vi "Dash Bools.vi"(1 "Input":cluster{"Arm Safety":bool, "Arm Limit":bool}, 2 "Menu":T1) -> (0 "Output":cluster{"Arm Safety":bool, "Arm Limit":bool})   [LabVIEW 2013]
uses:
  typedefs/fg_typedef.ctl
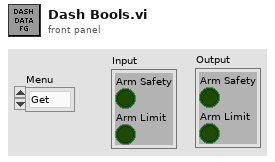
[diagram p1: front panel]
types:
  T1 = typedef "fg_typedef.ctl" = enum16{"Get", "Set"}
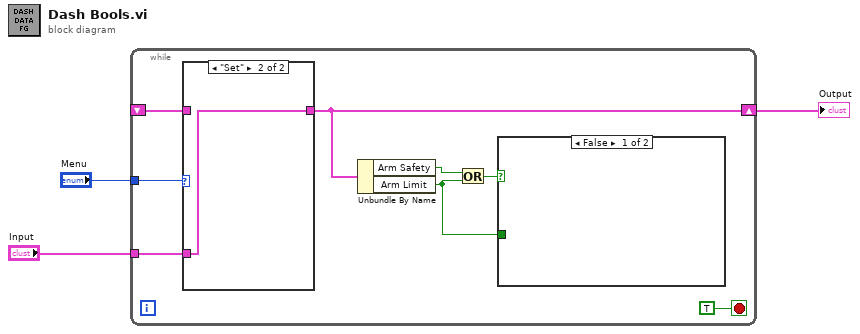
[diagram p0: block diagram]
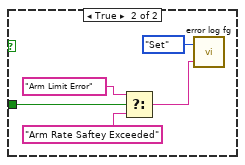
[diagram p2: hidden frame]
diagram:
  n1 = while {
    tunnel: "Menu" -> [w10]
    shift-right: [w7] -> w1
    shift-left: _ -> [w9]
    tunnel: "Input" -> [w8]
    stop <- TRUE stop-if-true
    n2 = case shown="\"Set\"" w10 {
      tunnel: w9 -> [w17 _]
      tunnel: [w17 w18] -> w7
      tunnel: w8 -> [_ w18]
      frame "Get", Default {
      }
      frame "Set" {
      }
    }
    n3 = Unbundle By Name(w7) -> ("Arm Safety"=w6:bool, "Arm Limit"=w4:bool)
    n4 = Or(x=w6, y=w4) -> (x .or. y?=w5:bool)
    n5 = case shown="False" w5 {
      tunnel: w4 -> [_ w15]
      frame False {
      }
      frame True {
        n6 = Select(t="Arm Limit Error", s=w15, f="Arm Rate Saftey Exceeded") -> (s? t:f=w12:string)
        n7 = call "error log fg.vi"("Error"=w12, "Log Mode"=enum16{"Get", "Set", "Clear"}."Set") -> ()  [unwired: 2 out]
      }
    }
  }
  "Output" <- w1
